vi "biref.vi"() -> ()   [LabVIEW 2021]
panel:
  in  "field increment":dbl
  out "Current field":dbl
  in  "Initial field T":dbl=0.08
  in  "No  Steps":i16
  out "outputdc 2":dbl[](array[numeric]) format="%.2f"
  in  "GPIB address dc meter 2":string="2"
  out "dup directory path":path
  in  "GPIB address dc meter":string="5"
  in  "GPIB  address  lockin":string="3"
  in  "GPIB address magnet":string="1"
  in  "GPIB address Temp controller":string="12"
  in  "Wait (second)":sgl
  in  "No of Temp Steps":i16
  in  "folder name to save files":string
  out "outputtemp":dbl[](array[numeric]) format="%.2f"
  out "outputdc":dbl[](array[numeric]) format="%.2f"
  out "outputlockin 2":dbl[](array[numeric]) format="%.2f"
  out "outputlockin 1":dbl[](array[numeric]) format="%.2f"
  out "field":dbl[](array[numeric]) format="%.2f"
  out "Current Temp":dbl format="%.3f"
  in  "Increasing \nTemp step":bool=TRUE
  in  "Initial Temp C":dbl format="%.3f"
  # "Help:\n1. write the folder name to save the files.The file name will \nbe the temperature in the given folder.\n2.Write the GPIB address of all the instruments before running\nthe program.\n3. Give the initial temperature and the temperature interval \nand the total number of steps.\n4.Check whether you want to increase the temperature or\ndecrease.\n5.Write the time to be waited to let the tempetature controller\nequilibrate.\n6.Once the speps 1 through 5 is done run the experiment."
  # "Decreasing\nTemp Step"
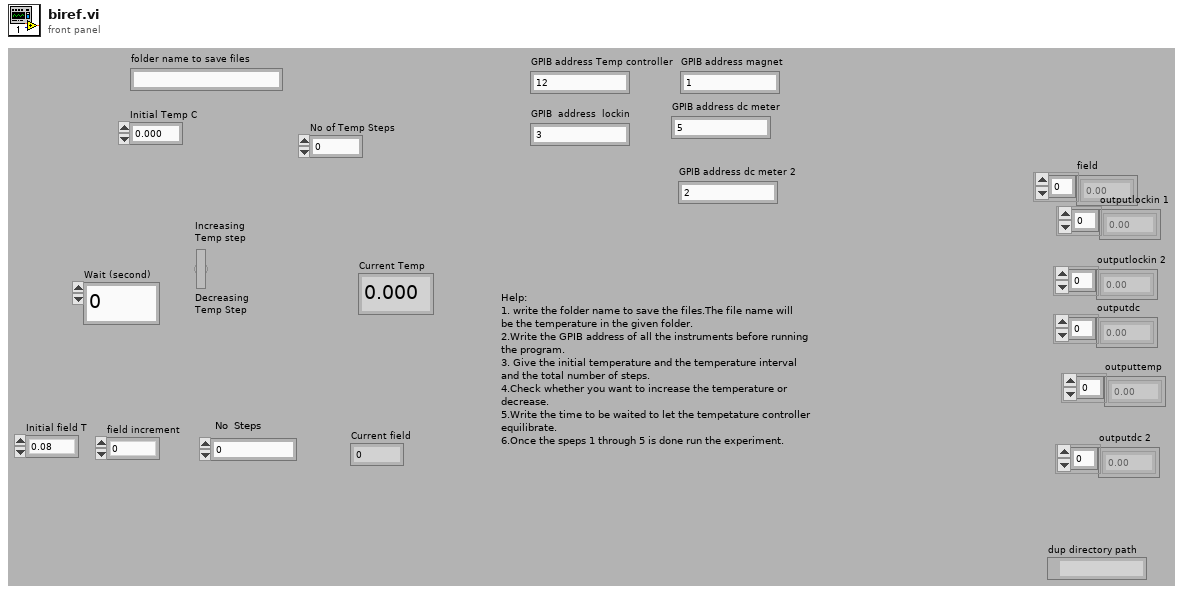
[diagram p1: front panel]
types:
  T1 = enum16{"--Quit--", "Read-Status", "Read-Cell", "Read-Field[T]", "Read-Setpoint[T]"}
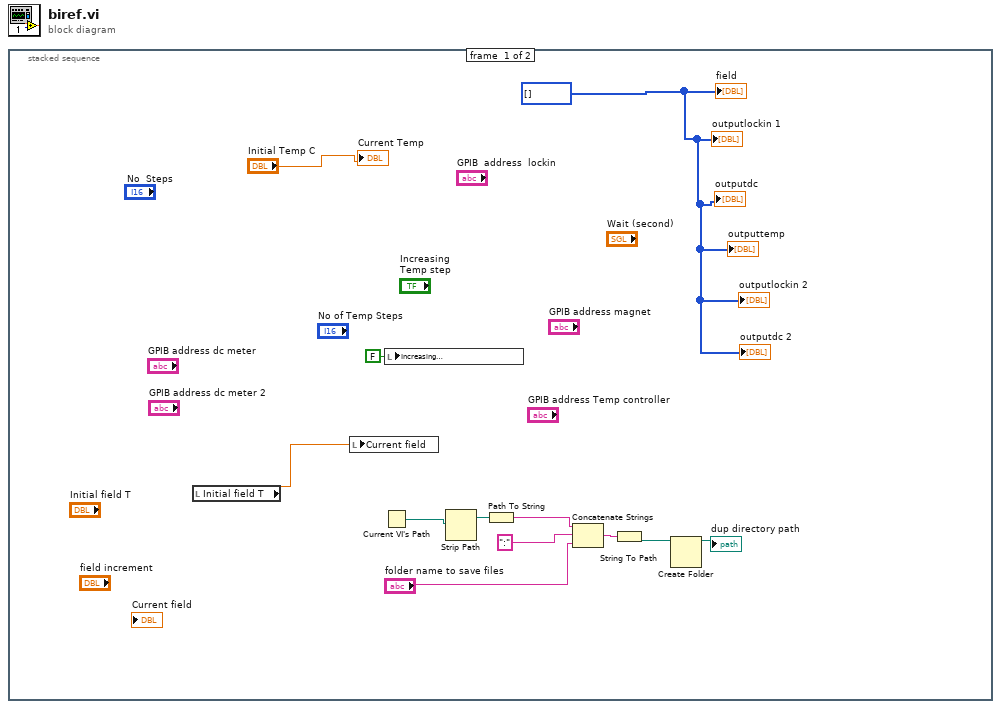
[diagram p0: block diagram]
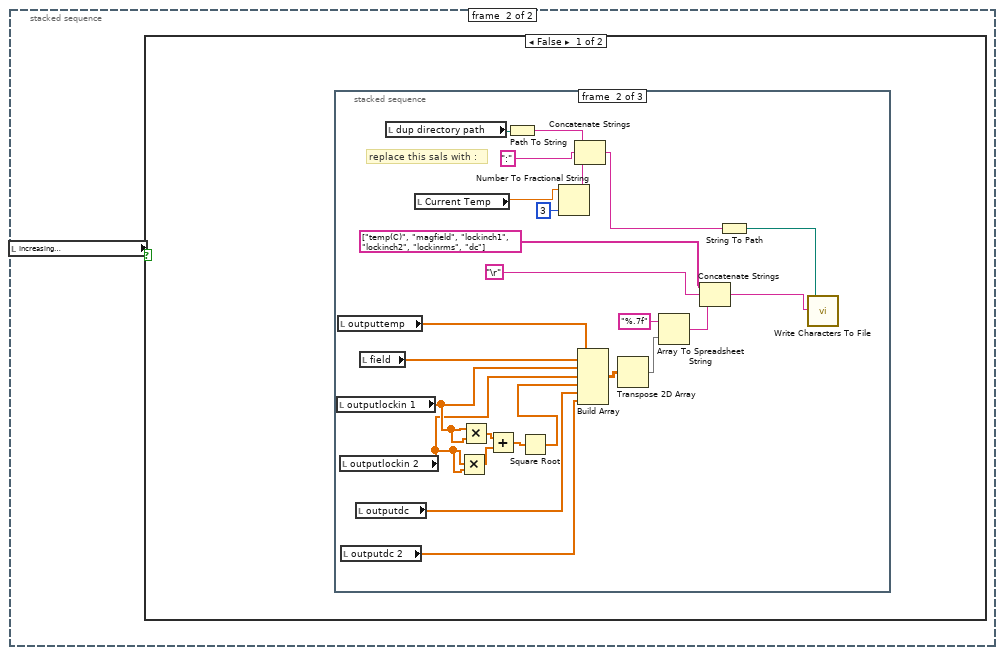
[diagram p2: hidden frame]
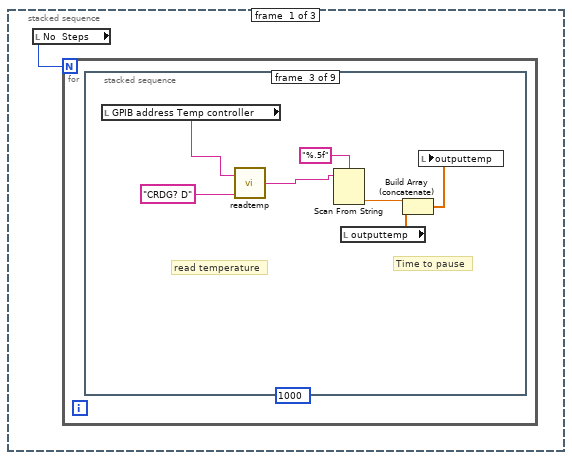
[diagram p3: hidden frame]
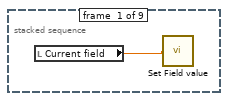
[diagram p4: hidden frame]
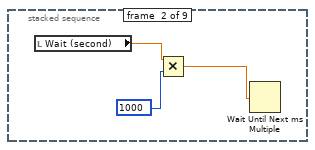
[diagram p5: hidden frame]
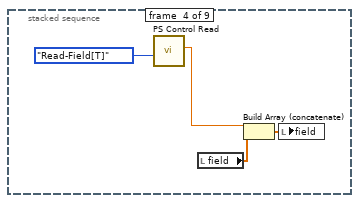
[diagram p6: hidden frame]
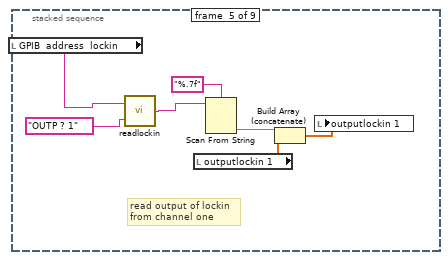
[diagram p7: hidden frame]
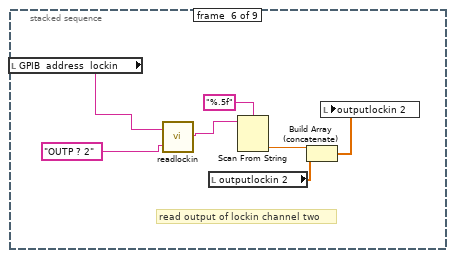
[diagram p8: hidden frame]
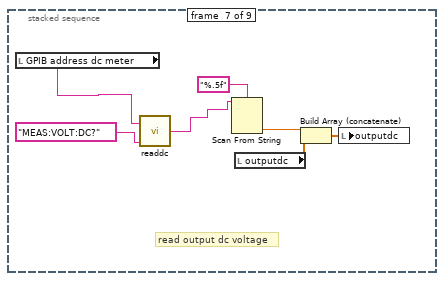
[diagram p9: hidden frame]
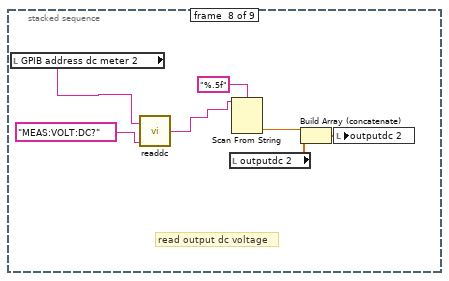
[diagram p10: hidden frame]
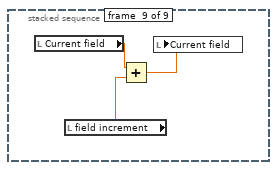
[diagram p11: hidden frame]
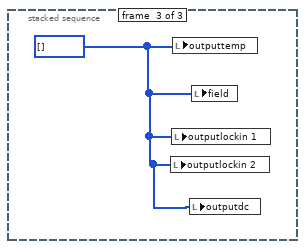
[diagram p12: hidden frame]
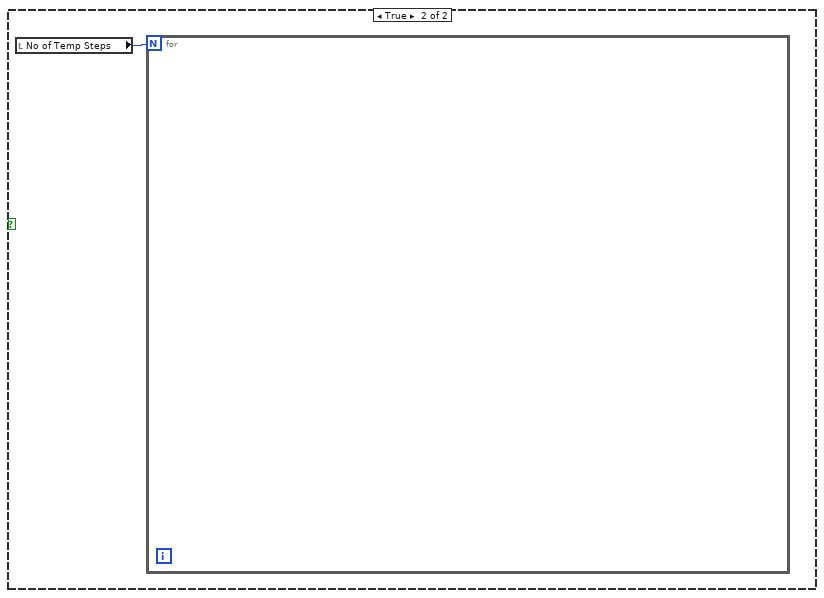
[diagram p13: hidden frame]
diagram:
  n1 = stacked-sequence {
    frame #0 {
      w3 = i32[] [] ("field")
      n2 = local read "Initial field T"() -> (w1:dbl)
      n3 = local write "Current field"(w1) -> ()
      n4 = Current VI's Path() -> (path=w11:path)
      n5 = local write "Increasing \nTemp step"(FALSE ("Increasing \nTemp step")) -> ()
      n6 = Strip Path(path=w11) -> (stripped path=w10:path)  [unwired: 1 out]
      n7 = Path To String(path=w10) -> (string=w9:string)
      n8 = Concatenate Strings(w9, ":", "folder name to save files") -> (w6:string)
      n9 = String To Path(string=w6) -> (path=w5:path)
      n10 = Create Folder(path (use dialog)=w5) -> (created path=→"dup directory path":path)  [unwired: 2 in, 2 out]
      "Current Temp" <- "Initial Temp C"
      "field" <- w3
      "outputlockin 1" <- w3
      "outputdc" <- w3
      "outputtemp" <- w3
      "outputlockin 2" <- w3
      "outputdc 2" <- w3
    }
    frame #1 {
      n11 = local read "Increasing \nTemp step"() -> (w13:bool)
      n12 = case shown="False" w13 {
        frame False {
          n13 = stacked-sequence {
            frame #0 {
              n14 = local read "No  Steps"() -> (w14:i16)
              n15 = for {
                N: w14 -> [_]
                n16 = stacked-sequence {
                  frame #0 {
                    n17 = local read "Current field"() -> (w15:dbl)
                    n18 = call "Set Field value.vi"("Field"=w15) -> ()
                  }
                  frame #1 {
                    n19 = local read "Wait (second)"() -> (w18:sgl)
                    n20 = Multiply(x=w18, y=u32 1000 ("millisecond multiple")) -> (x*y=w16:sgl)
                    n21 = Wait Until Next ms Multiple(millisecond multiple=w16) -> ()  [unwired: 1 out]
                  }
                  frame #2 {
                    (unwired) u32 1000 ("millisecond multiple")
                    # "Time to pause"
                    # "read temperature"
                    n22 = local read "GPIB address Temp controller"() -> (w19:string)
                    n23 = call "readtemp.vi"("Characters to Write"="CRDG? D", "GPIB\nAddress"=w19) -> ("Characters Read"=w20:string)
                    n24 = Scan From String(format string="%.5f", input string=w20) -> (output 1=w22:dbl)  [unwired: 3 in, 3 out]
                    n25 = local read "outputtemp"() -> (w25:dbl[])
                    n26 = Build Array (concatenate)(w22, w25) -> (w24:dbl[])
                    n27 = local write "outputtemp"(w24) -> ()
                  }
                  frame #3 {
                    n28 = call "PS Control Read.vi"("Read State"=T1."Read-Field[T]") -> ("Current Field"=w26:dbl)  [unwired: 3 in, 4 out]
                    n29 = local read "field"() -> (w28:dbl[])
                    n30 = Build Array (concatenate)(w26, w28) -> (w27:dbl[])
                    n31 = local write "field"(w27) -> ()
                  }
                  frame #4 {
                    # "read output of lockin\nfrom channel one"
                    n32 = local read "GPIB  address  lockin"() -> (w30:string)
                    n33 = call "readlockin.vi"("Characters to Write"="OUTP ? 1", "GPIB\nAddress"=w30) -> ("Characters Read"=w31:string)
                    n34 = local read "outputlockin 1"() -> (w35:dbl[])
                    n35 = Scan From String(format string="%.7f", input string=w31) -> (output 1=w32:dbl)  [unwired: 3 in, 3 out]
                    n36 = Build Array (concatenate)(w32, w35) -> (w34:dbl[])
                    n37 = local write "outputlockin 1"(w34) -> ()
                  }
                  frame #5 {
                    # "read output of lockin channel two"
                    n38 = local read "GPIB  address  lockin"() -> (w37:string)
                    n39 = call "readlockin.vi"("Characters to Write"="OUTP ? 2", "GPIB\nAddress"=w37) -> ("Characters Read"=w38:string)
                    n40 = local read "outputlockin 2"() -> (w42:dbl[])
                    n41 = Scan From String(format string="%.5f", input string=w38) -> (output 1=w40:dbl)  [unwired: 3 in, 3 out]
                    n42 = Build Array (concatenate)(w40, w42) -> (w41:dbl[])
                    n43 = local write "outputlockin 2"(w41) -> ()
                  }
                  frame #6 {
                    # "read output dc voltage"
                    n44 = local read "GPIB address dc meter"() -> (w44:string)
                    n45 = call "readdc.vi"("Characters to Write"="MEAS:VOLT:DC?", "GPIB\nAddress"=w44) -> ("Characters Read"=w45:string)
                    n46 = Scan From String(format string="%.5f", input string=w45) -> (output 1=w47:dbl)  [unwired: 3 in, 3 out]
                    n47 = local read "outputdc"() -> (w50:dbl[])
                    n48 = Build Array (concatenate)(w47, w50) -> (w49:dbl[])
                    n49 = local write "outputdc"(w49) -> ()
                  }
                  frame #7 {
                    # "read output dc voltage"
                    n50 = local read "GPIB address dc meter 2"() -> (w51:string)
                    n51 = call "readdc.vi"("Characters to Write"="MEAS:VOLT:DC?", "GPIB\nAddress"=w51) -> ("Characters Read"=w52:string)
                    n52 = local read "outputdc 2"() -> (w57:dbl[])
                    n53 = Scan From String(format string="%.5f", input string=w52) -> (output 1=w54:dbl)  [unwired: 3 in, 3 out]
                    n54 = Build Array (concatenate)(w54, w57) -> (w56:dbl[])
                    n55 = local write "outputdc 2"(w56) -> ()
                  }
                  frame #8 {
                    n56 = local read "Current field"() -> (w60:dbl)
                    n57 = local read "field increment"() -> (w59:dbl)
                    n58 = Add(x=w60, y=w59) -> (x+y=w58:dbl)
                    n59 = local write "Current field"(w58) -> ()
                  }
                }
              }
            }
            frame #1 {
              # "replace this sals with :"
              n60 = local read "outputlockin 1"() -> (w78:dbl[])
              n61 = local read "outputtemp"() -> (w80:dbl[])
              n62 = local read "outputlockin 2"() -> (w77:dbl[])
              n63 = local read "outputdc 2"() -> (w61:dbl[])
              n64 = local read "outputdc"() -> (w72:dbl[])
              n65 = local read "field"() -> (w79:dbl[])
              n66 = local read "dup directory path"() -> (w63:path)
              n67 = local read "Current Temp"() -> (w82:dbl)
              n68 = Multiply(x=w77, y=w77) -> (x*y=w75:dbl[])
              n69 = Multiply(x=w78, y=w78) -> (x*y=w76:dbl[])
              n70 = Add(x=w76, y=w75) -> (x+y=w74:dbl[])
              n71 = Path To String(path=w63) -> (string=w62:string)
              n72 = Square Root(x=w74) -> (sqrt(x)=w73:dbl[])
              n73 = Number To Fractional String(number=w82, precision (6)=i16 3) -> (F-format string=w81:string)  [unwired: 2 in]
              n74 = Concatenate Strings(w62, ":", w81) -> (w84:string)
              n75 = Build Array(w80, w79, w78, w77, w73, w72, w61) -> (w71:dbl[][])
              n76 = Transpose 2D Array(2D array=w71) -> (transposed array=w69:dbl[][])
              n77 = Array To Spreadsheet String(array=w69, 3:"%.7f" ("format string")) -> (spreadsheet string=w66:string)  [unwired: 1 in]
              n78 = Concatenate Strings(string[] ["temp(C)", "magfield", "lockinch1", "lockinch2", "lockinrms", "dc"], "\r", w66) -> (w65:string)
              n79 = String To Path(string=w84) -> (path=w83:path)
              n80 = call <vilib>:"Write Characters To File.vi"("character string"=w65, "file path (dialog if empty)"=w83) -> ()  [unwired: 3 in, 1 out]
            }
            frame #2 {
              w86 = i32[] []
              n81 = local write "outputlockin 2"(w86) -> ()
              n82 = local write "outputlockin 1"(w86) -> ()
              n83 = local write "outputtemp"(w86) -> ()
              n84 = local write "outputdc"(w86) -> ()
              n85 = local write "field"(w86) -> ()
            }
          }
        }
        frame True {
          n86 = local read "No of Temp Steps"() -> (w87:i16)
          n87 = for {
            N: w87 -> [_]
          }
        }
      }
    }
  }
